vi "Protocol.Claim Addresses.vi"(8 "error in":errorcluster, 10 "Parameters in":T16={"Name"="", "XNET.Settings"={"Database"="", "Cluster"="", "Port"="", "Baud rate [Bd]"=0, "Termination"=0, "Incoming Decimation"=0, "Outgoing Decimation"=1}, "Monitor.Network"={"Address"=0, "Name"=0, "Include DA"=FALSE}, "Data"=[], "DTCs"=[], "Sim.Nodes.LUT"=variant, "Data.LUT"=variant, "PCL"=0} {"Monitor.Network"."Name" format="%.0x"; "DTCs"."Data"."DM1.Ref"."Data Reference" format="%.0x"; "DTCs"."Data"."DM1.Enable.Ref"."Data Reference" format="%.0x"; "DTCs"."Data"."DM2.Ref"."Data Reference" format="%.0x"; "DTCs"."Data"."DM2.Enable.Ref"."Data Reference" format="%.0x"; "Data"."Trigger.Refs"."Data Reference" format="%.0x"; "Data"."Disable.Refs"."Data Reference" format="%.0x"; "Data"."Timing.Refs"."Data Reference" format="%.0x"; "Data"."Network"."Name" format="%.0x"; "Data"."Incoming.Refs"."Data Reference" format="%.0x"; "Data"."Outgoing.Refs"."Data Reference" format="%.0x"; "XNET.Settings"."Termination" items=["Off", "On"]}, 11 "J1939 Main Configuration":T1) -> (0 "error out":errorcluster, 3 "output cluster":T1)   [LabVIEW 2019, in "J1939 Addon Engine.lvlib"]
uses:
  J1939 Addon Engine.lvlib
  Types/Protocol.Configuration.ctl
  <vilib>/NI/NI VeriStand Addon Network Comm/Engine/VeriStand Comm.lvclass
  <vilib>/NI/NIVS Inline Async API/_VS Inline Async API/Process/Process.lvclass
  Types/Protocol.Refs.ctl
  Support Libraries/J1939 Utilities/Types/CAN Outgoing Message Cluster.ctl
  Types/Protocol.RQST Lookup Table Reference.ctl
  Types/Protocol.Address Table Reference.ctl
  Types/Protocol.XNET Settings.ctl
  <vilib>/NI/NIVS Inline Async API/_Data Access Engine/Data Access Engine/Types/Read.DVR.ctl
  <vilib>/NI/NIVS Inline Async API/_Data Access Engine/Access Type Classes/Read/Read.lvclass
  <vilib>/NI/NIVS Inline Async API/_Data Access Engine/Data Access Engine/Types/Write.DVR.ctl
  <vilib>/NI/NIVS Inline Async API/_Data Access Engine/Access Type Classes/Write/Write.lvclass
  Types/CounterAndProtectionFrames.ctl
  SubModules/Frame Protection Support/Source/Engine/Types/RT Frame Settings.ctl
  SubModules/Frame Protection Support/Source/Shared/Types/Exported Frame Type.ctl
  SubModules/Frame Protection Support/Source/Engine/Types/RT Protection Configuration.ctl
  SubModules/Frame Protection Support/Source/Shared/Types/Protection Type.ctl
  SubModules/Frame Protection Support/Source/Shared/Types/XNET Signal Configuration.ctl
  SubModules/Frame Protection Support/Source/Shared/Types/Exported Counter Settings.ctl
  SubModules/Frame Protection Support/Source/Shared/Types/Exported Event Trigger Type.ctl
  Types/Protocol.App Settings.ctl
  Addon Shared/Types/XNET Settings.ctl
  Addon Shared/Types/Monitor Settings.ctl
  Types/Protocol.XNET Refs.ctl
  <vilib>/NI VeriStand/Custom Device API/Block Data Reference.ctl
  <vilib>/NI VeriStand/Custom Device API/Data Reference.ctl
  Types/Main.Outgoing.Frame.Settings.ctl
  Addon Shared/Types/Outgoing Event Trigger Types.ctl
  SubModules/Frame Protection Support/Source/Shared/Types/Exported Frame Settings.ctl
  SubModules/Frame Protection Support/Source/Shared/Types/Exported Protection Settings.ctl
  Types/Engine.DTC Settings.ctl
  Addon Shared/Types/Compiled Simulated Settings.ctl
  Types/Engine.DTC FIFOs.ctl
  <vilib>/Utility/SystemLogging/Write to System Log.vi
  <resource>/objmgr/xnet.rc
  Support Libraries/J1939 Utilities/J1939 Utilities.lvlib
  Addon Shared/J1939 Addon Shared.lvlib
  <vilib>/NI VeriStand/Custom Device API/Custom Device API.lvlib
  <vilib>/NI/NIVS Inline Async API/_Data Access Engine/Data Access Engine/Data Access Engine.lvclass
  SubModules/Frame Protection Support/Source/Engine/Protection and Counter Support Engine.lvlib
  SubModules/Frame Protection Support/Source/Shared/Protection and Counter Support Shared.lvlib
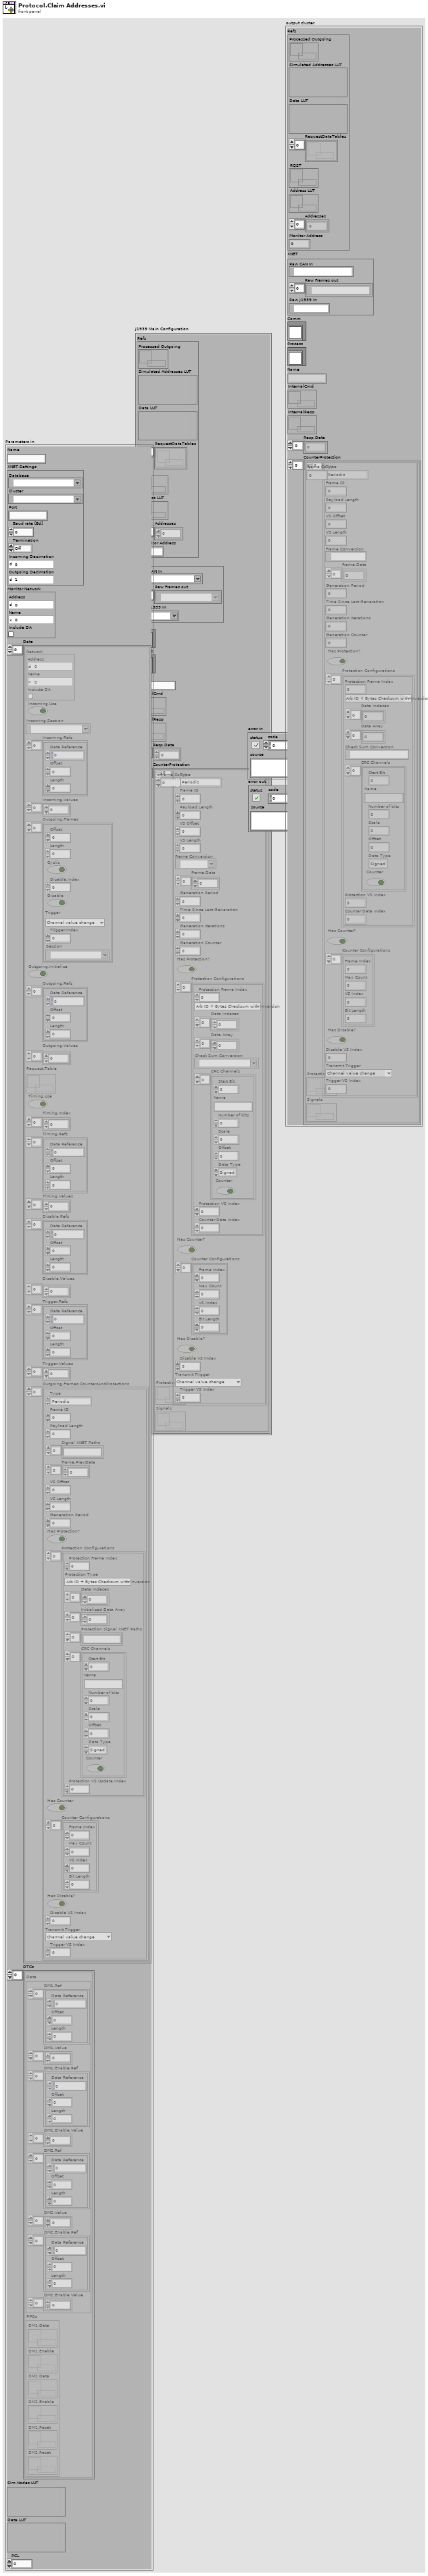
[diagram p1: front panel]
types:
  T1 = typedef "J1939 Addon Engine.lvlib/Protocol.Configuration.ctl" = cluster{"Refs":T2, "XNET":T5, "Comm":refnum<class "VeriStand Comm.lvclass">, "Process":refnum<class "Process.lvclass">, "Name":string, "InternalCmd":T6, "InternalResp":T7, "Resp.Data":dbl[], "CounterProtection":T8[]}
  T2 = typedef "J1939 Addon Engine.lvlib/Protocol.Refs.ctl" = cluster{"Processed Outgoing":refnum<queue>, "Simulated Addresses LUT":variant, "Data LUT":variant, "RequestDataTables":refnum<k33>[], "RQST":T3, "Address LUT":T4, "Addresses":u8[], "Monitor Address":u8}
  T3 = typedef "J1939 Addon Engine.lvlib/Protocol.RQST Lookup Table Reference.ctl" = refnum<data-value>
  T4 = typedef "J1939 Addon Engine.lvlib/Protocol.Address Table Reference.ctl" = refnum<data-value>
  T5 = typedef "J1939 Addon Engine.lvlib/Protocol.XNET Settings.ctl" = cluster{"Raw CAN In":refnum<k21>, "Raw Frames out":refnum<k21>[], "Raw J1939 In":refnum<k21>}
  T6 = typedef "Data Access Engine.lvlib/Data Access Engine.lvclass/Read.DVR.ctl" = refnum<data-value>
  T7 = typedef "Data Access Engine.lvlib/Data Access Engine.lvclass/Write.DVR.ctl" = refnum<data-value>
  T8 = typedef "J1939 Addon Engine.lvlib/CounterAndProtectionFrames.ctl" = cluster{"Frame Count":i32, "Frames in":T9[], "Protections":T7, "Signals":T6}
  T9 = typedef "Protection and Counter Support Engine.lvlib/RT Frame Settings.ctl" = cluster{"Type":T10, "Frame ID":u32, "Payload Length":u32, "VS Offset":i32, "VS Length":i32, "Frame Conversion":refnum<k21>, "Frame.Data":dbl[], "Generation Period":u32, "Time Since Last Generation":u32, "Generation Iterations":u32, "Generation Counter":u32, "Has Protection?":bool, "Protection Configurations":T11[], "Has Counter?":bool, "Counter Configurations":T14[], "Has Disable?":bool, "Disable VS Index":i32, "Transmit Trigger":T15, "Trigger VS Index":i32}
  T10 = typedef "Protection and Counter Support Shared.lvlib/Exported Frame Type.ctl" = enum16{"Periodic", "Event", "Periodic/Event"}
  T11 = typedef "Protection and Counter Support Engine.lvlib/RT Protection Configuration.ctl" = cluster{"Protection Frame Index":i32, "Protection Type":T12, "Data Indeces":i32[], "Data Array":dbl[], "Check Sum Conversion":refnum<k21>, "CRC Channels":T13[], "Protection VS Index":i32, "Counter Data Index":i32}
  T12 = typedef "Protection and Counter Support Shared.lvlib/Protection Type.ctl" = enum16{"Arb ID + Bytes Checksum with Inversion", "Arb ID + Bytes CRC with Inversion", "Reversed Raw Signal Checksum with Inversion", "Concatenated Two's Compliment"}
  T13 = typedef "Protection and Counter Support Shared.lvlib/XNET Signal Configuration.ctl" = cluster{"Start Bit":i32, "Name":string, "Number of bits":i32, "Scale":dbl, "Offset":dbl, "Data Type":u32, "Counter":bool}
  T14 = typedef "Protection and Counter Support Shared.lvlib/Exported Counter Settings.ctl" = cluster{"Frame Index":i32, "Max Count":dbl, "VS Index":i32, "Bit Length":i64}
  T15 = typedef "Protection and Counter Support Shared.lvlib/Exported Event Trigger Type.ctl" = enum16{"Channel value change", "Trigger channel (not zero)", "Channel value change or trigger channel (not zero)", "Trigger channel (any value change)", "Channel value change or trigger channel (any value change)"}
  T16 = typedef "J1939 Addon Engine.lvlib/Protocol.App Settings.ctl" = cluster{"Name":string, "XNET.Settings":T17, "Monitor.Network":T18, "Data":T19[], "DTCs":T26[], "Sim.Nodes.LUT":variant, "Data.LUT":variant, "PCL":u32}
  T17 = typedef "J1939 Addon Shared.lvlib/XNET Settings.ctl" = cluster{"Database":refnum<k21>, "Cluster":refnum<k21>, "Port":string, "Baud rate [Bd]":u32, "Termination":u32, "Incoming Decimation":u32, "Outgoing Decimation":u32}
  T18 = typedef "J1939 Addon Shared.lvlib/Monitor Settings.ctl" = cluster{"Address":u8, "Name":u64, "Include DA":bool}
  T19 = typedef "J1939 Addon Engine.lvlib/Protocol.XNET Refs.ctl" = cluster{"Network":T18, "Incoming.Use":bool, "Incoming.Session":refnum<k21>, "Incoming.Refs":T20[], "Incoming.Values":dbl[], "Outgoing.Frames":T22[], "Outgoing.Initialize":bool, "Outgoing.Refs":T20[], "Outgoing.Values":dbl[], "Request.Table":refnum<k33>, "Timing.Use":bool, "Timing.Index":i32[], "Timing.Refs":T20[], "Timing.Values":dbl[], "Disable.Refs":T20[], "Disable.Values":dbl[], "Trigger.Refs":T20[], "Trigger.Values":dbl[], "Outgoing.Frames.CountersAndProtections":T24[]}
  T20 = typedef "Custom Device API.lvlib/Block Data Reference.ctl" = cluster{"Data Reference":T21, "Offset":u64, "Length":u64}
  T21 = typedef "Custom Device API.lvlib/Data Reference.ctl" = i32
  T22 = typedef "J1939 Addon Engine.lvlib/Main.Outgoing.Frame.Settings.ctl" = cluster{"Offset":u32, "Length":u32, "Cyclic":bool, "Disable.Index":i32, "Disable":bool, "Trigger":T23, "Trigger.Index":i32, "Session":refnum<k21>}
  T23 = typedef "J1939 Addon Shared.lvlib/Outgoing Event Trigger Types.ctl" = enum16{"Channel value change", "Trigger channel (not zero)", "Channel value change or trigger channel (not zero)", "Trigger channel (any value change)", "Channel value change or trigger channel (any value change)"}
  T24 = typedef "Protection and Counter Support Shared.lvlib/Exported Frame Settings.ctl" = cluster{"Type":T10, "Frame ID":u32, "Payload Length":u32, "Signal XNET Paths":string[], "Frame.PrevData":dbl[], "VS Offset":i32, "VS Length":i32, "Generation Period":u32, "Has Protection?":bool, "Protection Configurations":T25[], "Has Counter":bool, "Counter Configurations":T14[], "Has Disable?":bool, "Disable VS Index":i32, "Transmit Trigger":T15, "Trigger VS Index":i32}
  T25 = typedef "Protection and Counter Support Shared.lvlib/Exported Protection Settings.ctl" = cluster{"Protection Frame Index":i32, "Protection Type":T12, "Data Indeces":i32[], "Initialized Data Array":dbl[], "Protection Signal XNET Paths":string[], "CRC Channels":T13[], "Protection VS Update Index":i32}
  T26 = typedef "J1939 Addon Engine.lvlib/Engine.DTC Settings.ctl" = cluster{"Data":T27, "FIFOs":T28}
  T27 = typedef "J1939 Addon Shared.lvlib/Compiled Simulated Settings.ctl" = cluster{"DM1.Ref":T20[], "DM1.Value":dbl[], "DM1.Enable.Ref":T20[], "DM1.Enable.Value":dbl[], "DM2.Ref":T20[], "DM2.Value":dbl[], "DM2.Enable.Ref":T20[], "DM2.Enable.Value":dbl[]}
  T28 = typedef "J1939 Addon Engine.lvlib/Engine.DTC FIFOs.ctl" = cluster{"DM1.Data":refnum<k33>, "DM1.Enable":refnum<k33>, "DM2.Data":refnum<k33>, "DM2.Enable":refnum<k33>, "DM1.Reset":refnum<k33>, "DM2.Reset":refnum<k33>}
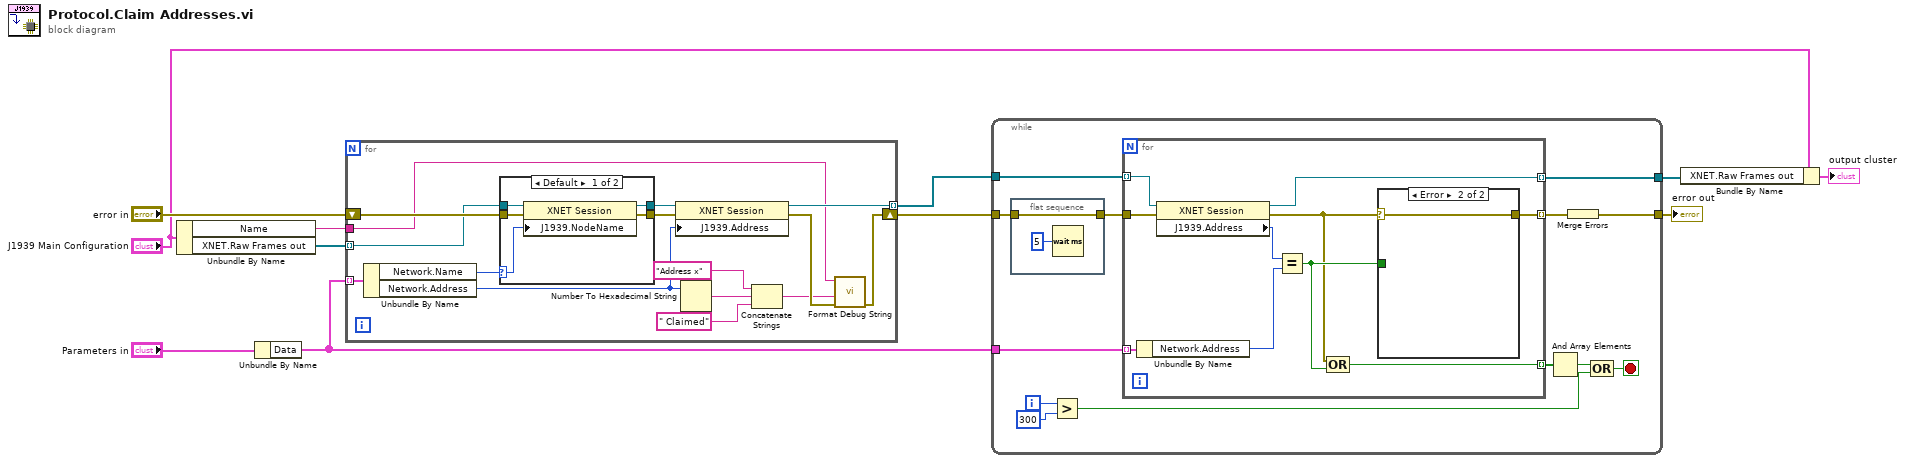
[diagram p0: block diagram]
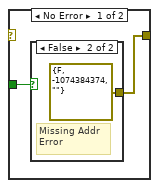
[diagram p2: hidden frame]
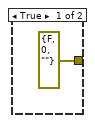
[diagram p3: hidden frame]
diagram:
  n1 = Unbundle By Name("J1939 Main Configuration") -> ("Name"=w1:string, "XNET.Raw Frames out"=w9:refnum<k21>[])
  n2 = Unbundle By Name("Parameters in") -> ("Data"=w7:T19[])
  n3 = for {
    shift-right: [w15] -> w11
    shift-left: "error in" -> [w26]
    tunnel: w7 -> [w23] mode=indexing
    tunnel: w9 -> [w21] mode=indexing
    tunnel: [w20] -> w10 mode=indexing
    tunnel: w1 -> [w12]
    n4 = Unbundle By Name(w23) -> ("Network.Name"=w22:u64, "Network.Address"=w19:u8)
    n5 = case shown="Default" w22 {
      selector: w22 -> [w29 _]
      tunnel: w21 -> [w31 w32]
      tunnel: w26 -> [w30 w33]
      tunnel: [w28 w33] -> w25
      tunnel: [w27 w32] -> w24
      frame Default {
        n6 = property class="XNET Session"(reference=w31, error in=w30, "J1939.NodeName"=w29) -> (reference out=w27:refnum<k21>, error out=w28:errorcluster)
      }
      frame 0 {
      }
    }
    n7 = property class="XNET Session"(reference=w24, error in=w25, "J1939.Address"=w19) -> (reference out=w20:refnum<k21>, error out=w16:errorcluster)
    n8 = Number To Hexadecimal String(2:w19) -> (0:w18:string)  [unwired: 1 in]
    n9 = Concatenate Strings("Address x" ("Message"), w18, " Claimed" ("string")) -> (w14:string)
    n10 = call "Format Debug String.vi"("error in (no error)"=w16, "State"=w14, "Name"=w12) -> ("error out"=w15:errorcluster)  [unwired: 8 in]
  }
  n11 = while {
    tunnel: w11 -> [w43]
    tunnel: [w45] -> w5
    tunnel: w10 -> [w35]
    tunnel: w7 -> [w36]
    tunnel: [w34] -> w3
    i -> [w41]
    stop <- w37 stop-if-true
    n12 = flat-sequence {
      tunnel: [w48] -> w44
      tunnel: w43 -> [w48]
      frame #0 {
        n13 = Wait (ms)(milliseconds to wait=u32 5) -> ()  [unwired: 1 out]
      }
    }
    n14 = Greater?(x=w41, y=300) -> (0:w38:bool)
    n15 = for {
      tunnel: w44 -> [w58]
      tunnel: [w57] -> w46 mode=indexing
      tunnel: w35 -> [w56] mode=indexing
      tunnel: [w55] -> w40 mode=indexing
      tunnel: w36 -> [w54] mode=indexing
      tunnel: [w49] -> w34 mode=indexing
      n16 = Unbundle By Name(w54) -> ("Network.Address"=w53:u8)
      n17 = property class="XNET Session"(reference=w56, error in=w58) -> (reference out=w49:refnum<k21>, error out=w51:errorcluster, "J1939.Address"=w50:u8)
      n18 = Equal?(x=w50, y=w53) -> (x = y?=w52:bool)
      n19 = Compound Arithmetic op=OR(w51, w52) -> (w55:bool)
      n20 = case shown="Error" w51 {
        selector: w51 -> [_ w63]
        tunnel: w52 -> [w60 _]
        tunnel: [w59 w63] -> w57
        frame No Error {
          n21 = case shown="False" w60 {
            tunnel: [errorcluster {"status"=FALSE, "code"=0, "source"=""} ("error out") errorcluster {"status"=FALSE, "code"=-1074384374, "source"=""} ("error out")] -> w59
            frame True {
            }
            frame False {
              # "Missing Addr\nError"
            }
          }
        }
        frame Error {
        }
      }
    }
    n22 = And Array Elements(Boolean array=w40) -> (logical AND=w39:bool)
    n23 = Merge Errors(w46) -> (w45:errorcluster)
    n24 = Compound Arithmetic op=OR(w39, w38) -> (w37:bool)
  }
  "error out" <- w5
  n25 = Bundle By Name(cluster="J1939 Main Configuration", "XNET.Raw Frames out"=w3) -> (→"output cluster":T1)
